vi "PublishChannelNames.vi"(8 "error in (no error)":errorcluster, 9 "names":string[](array[string]), 10 "Qbus in":refnum<class "Qbus.lvclass">, 11 "config in":T1) -> (0 "error out":errorcluster, 3 "config out":T1)   [LabVIEW 2017, in "TestPanel.lvlib"]
uses:
  <vilib>/addons/InsightCM/Devices/Shared/Common/TestPanel/TestPanel.lvlib
  <vilib>/addons/InsightCM/Devices/Shared/Common/TestPanel/controls/Configuration.ctl
  <vilib>/addons/InsightCM/Devices/Shared/Common/TestPanel/controls/State.ctl
  <vilib>/addons/InsightCM/MessageBus/Base/controls/IRoutingSource.ctl
  <vilib>/addons/Qbus/Qbus.lvclass
  <vilib>/addons/InsightCM/MessageBus/MessageLibrary/Device/controls/DeviceTestPanelGetChannelNamesResponseBody.ctl
  <vilib>/addons/InsightCM/Devices/Shared/Common/ServerComm/ServerComm.lvlib
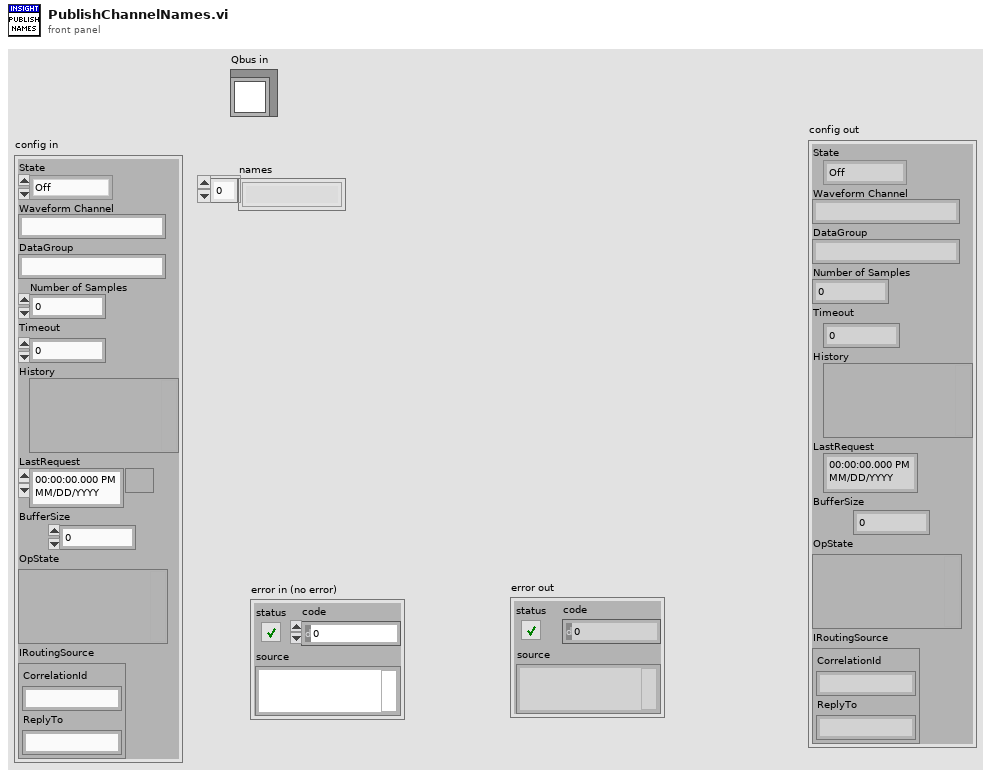
[diagram p1: front panel]
types:
  T1 = typedef "TestPanel.lvlib/Configuration.ctl" = cluster{"State":T2, "Waveform Channel":string, "DataGroup":string, "Number of Samples":i32, "Timeout":dbl, "History":variant, "LastRequest":timestamp, "BufferSize":i32, "OpState":variant, "IRoutingSource":T3}
  T2 = typedef "TestPanel.lvlib/State.ctl" = enum16{"Off", "On", "PendingValues", "PendingDataSet"}
  T3 = typedef "IRoutingSource.ctl" = cluster{"CorrelationId":string, "ReplyTo":string}
  T4 = typedef "DeviceTestPanelGetChannelNamesResponseBody.ctl" = cluster{"ChannelNames":string[]}
  T5 = typedef "Message.ctl" = cluster{"Header":T6, "Body":u8[]}
  T6 = typedef "MessageHeader.ctl" = cluster{"MessageName":string, "Timestamp":i64, "CorrelationId":string, "ContentType":string, "RoutingKey":string, "Properties":T7[]}
  T7 = typedef "KeyValuePair.ctl" = cluster{"Key":string, "Value":string}
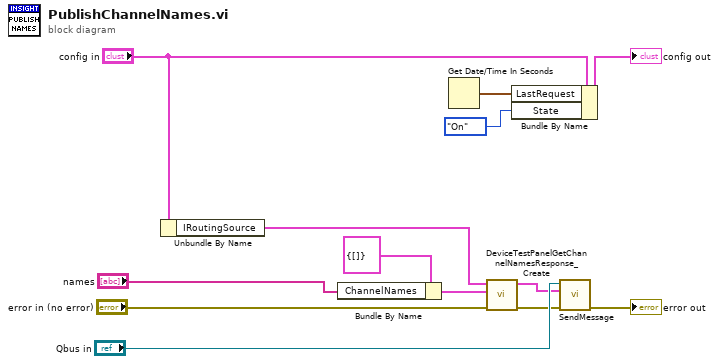
[diagram p0: block diagram]
diagram:
  n1 = Unbundle By Name("config in") -> ("IRoutingSource"=w7:T3)
  n2 = Bundle By Name(cluster=T4 {"ChannelNames"=[]} ("DeviceTestPanelGetChannelNamesResponse"), "ChannelNames"="names") -> (w3:T4)
  n3 = Get Date/Time In Seconds() -> (seconds since 1Jan1904=w11:timestamp)
  n4 = call <vilib>:"DeviceTestPanelGetChannelNamesResponse_Create.vi"("error in (no error)"="error in (no error)", "DeviceTestPanelGetChannelNamesResponse"=w3, "IRoutingSource"=w7) -> ("error out"=w5:errorcluster, "Message"=w6:T5)  [unwired: 7 in]
  n5 = Bundle By Name(cluster="config in", "LastRequest"=w11, "State"=State."On") -> (→"config out":T1)
  n6 = call <vilib>:"SendMessage.vi"("error in (no error)"=w5, "message"=w6, "Qbus in"="Qbus in") -> ("error out"=→"error out":errorcluster)  [unwired: 7 in, 1 out]
